vi "set properties for a control in a cluster using reference.vi"(8 "data entry":T1, 9 "type":string, 10 "name":string, 11 "Clust Refnum":refnum<vi>) -> ()   [LabVIEW 2015]
uses:
  <vilib>/Utility/miscctls.llb/LVOutOfRangeActionTypeDef.ctl
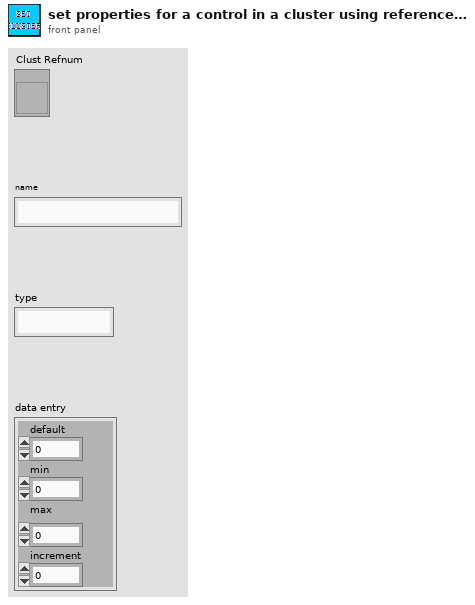
[diagram p1: front panel]
types:
  T1 = cluster{"default":dbl, "min":dbl, "max":dbl, "increment":dbl}
  T2 = typedef "LVOutOfRangeActionTypeDef.ctl" = cluster{"Out of Range Action Minimum":u8, "Out of Range Action Maximum":u8, "Out of Range Action Increment":u8}
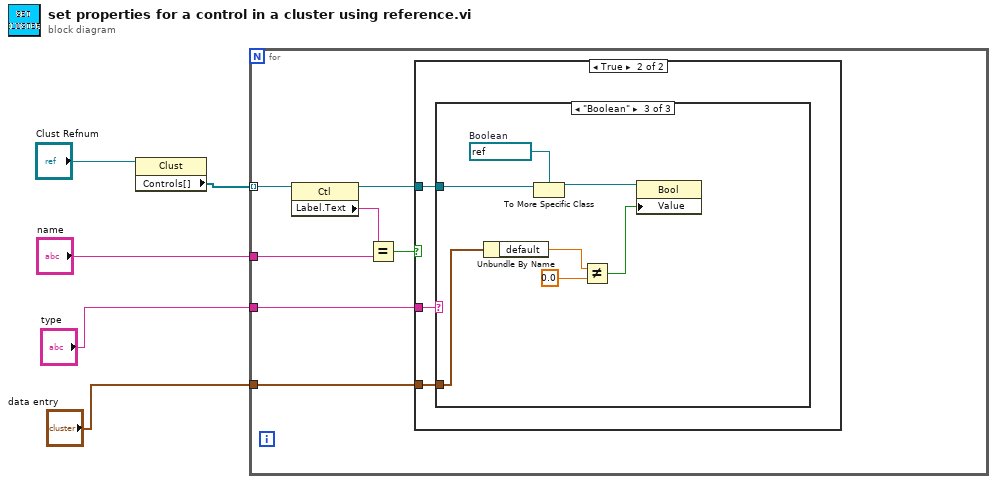
[diagram p0: block diagram]
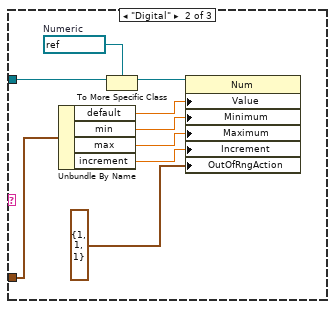
[diagram p4: hidden frame]
diagram:
  n1 = property class="Clust"(reference="Clust Refnum") -> ("Controls[]"=w4:refnum<vi>[])  [unwired: 1 in, 2 out]
  n2 = for {
    tunnel: w4 -> [w12] mode=indexing
    tunnel: "name" -> [w10]
    tunnel: "type" -> [w7]
    tunnel: "data entry" -> [w6]
    n3 = property class="Ctl"(reference=w12) -> (reference out=w8:refnum<vi>, "Label.Text"=w11:string)  [unwired: 1 in, 1 out]
    n4 = Equal?(x=w11, y=w10) -> (x = y?=w9:bool)
    n5 = case shown="True" w9 {
      tunnel: w8 -> [_ w14]
      tunnel: w7 -> [_ w15]
      tunnel: w6 -> [_ w13]
      frame False {
      }
      frame True {
        n6 = case shown="\"Boolean\"" w15 {
          tunnel: w14 -> [_ w24 w31]
          tunnel: w13 -> [_ w21 w28]
          frame "False", Default {
          }
          frame "Digital" {
            w23 = refnum<vi> refnum  # Numeric
            n7 = Unbundle By Name(w21) -> ("default"=w16:dbl, "min"=w17:dbl, "max"=w18:dbl, "increment"=w19:dbl)
            n8 = To More Specific Class(target class=w23, reference=w24) -> (specific class reference=w22:refnum<vi>)  [unwired: 1 in, 1 out]
            n9 = property class="Num"(reference=w22, "Value"=w16, "Minimum"=w17, "Maximum"=w18, "Increment"=w19, "OutOfRngAction"=T2 {"Out of Range Action Minimum"=1, "Out of Range Action Maximum"=1, "Out of Range Action Increment"=1} ("Response to Value Outside Limits")) -> ()  [unwired: 1 in, 2 out]
          }
          frame "Boolean" {
            w30 = refnum<vi> refnum  # Boolean
            n10 = Unbundle By Name(w28) -> ("default"=w26:dbl)
            n11 = To More Specific Class(target class=w30, reference=w31) -> (specific class reference=w29:refnum<vi>)  [unwired: 1 in, 1 out]
            n12 = Not Equal?(x=w26, y=0.0) -> (x != y?=w25:bool)
            n13 = property class="Bool"(reference=w29, "Value"=w25) -> ()  [unwired: 1 in, 2 out]
          }
        }
      }
    }
  }
